vi "SELECT SALES TRACKING COLUMNS.vi"(8 "Search Database Results":refnum<vi>, 9 "DATA IN":string[][](array[string]), 11 "Sales Tracking Column Selector":T1={"SALE ID #"=TRUE, "BYU ID CARD #"=TRUE, "Sale Description"=TRUE, "Grand Total"=TRUE, "SALE DATE"=TRUE, "ITEM DESCRIPTION"=TRUE, "ITEM QUANTITY"=TRUE, "ITEM UNIT PRICE"=TRUE, "ITEM TOTAL PRICE"=TRUE, "SALE SEMESTER"=TRUE}) -> (1 "HEADERS OUT":string[](array[string]), 3 "DATA OUT":string[][](array[string]))   [LabVIEW 2019]
uses:
  Controls/Column Names/Sales Tracking Column Names.ctl
  <vilib>/Utility/miscctls.llb/LVRowAndColumnTypeDef.ctl
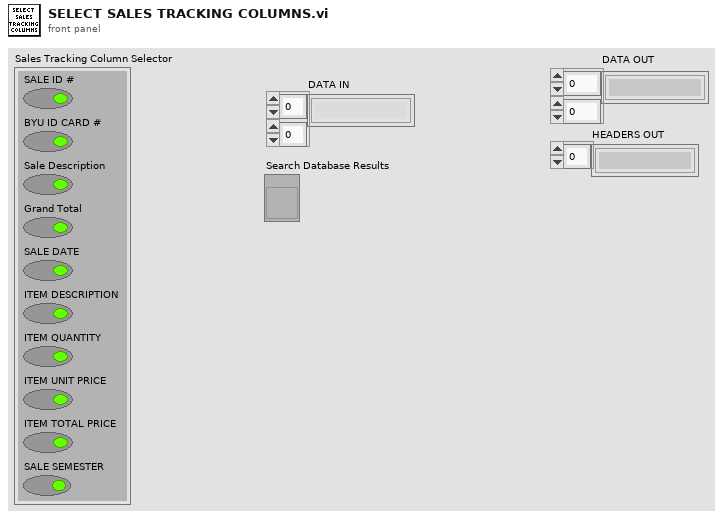
[diagram p1: front panel]
types:
  T1 = cluster{"SALE ID #":bool, "BYU ID CARD #":bool, "Sale Description":bool, "Grand Total":bool, "SALE DATE":bool, "ITEM DESCRIPTION":bool, "ITEM QUANTITY":bool, "ITEM UNIT PRICE":bool, "ITEM TOTAL PRICE":bool, "SALE SEMESTER":bool}
  T2 = typedef "Sales Tracking Column Names.ctl" = string[]
  T3 = typedef "LVRowAndColumnTypeDef.ctl" = cluster{"Row":i32, "Column":i32}
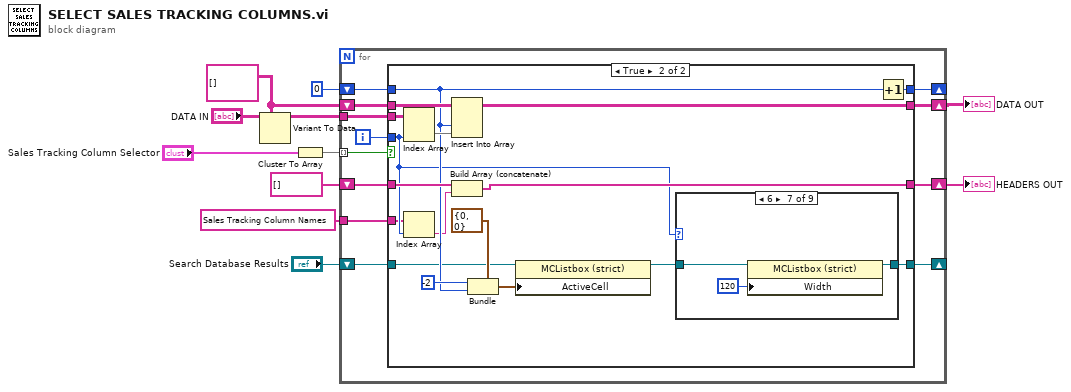
[diagram p0: block diagram]
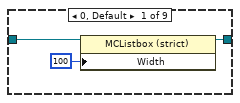
[diagram p3: hidden frame]
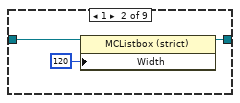
[diagram p4: hidden frame]
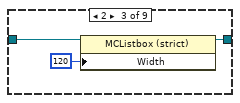
[diagram p5: hidden frame]
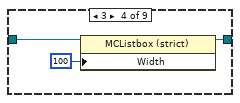
[diagram p6: hidden frame]
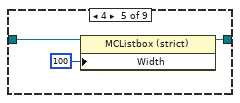
[diagram p7: hidden frame]
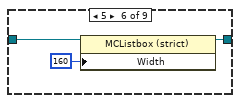
[diagram p8: hidden frame]
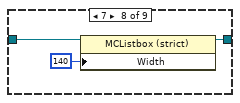
[diagram p9: hidden frame]
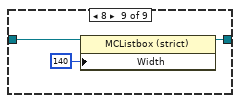
[diagram p10: hidden frame]
diagram:
  w7 = string[][] [] ("DATA OUT")
  n1 = Variant To Data(type=w7, Variant="DATA IN") -> (data=w8:string[][])  [unwired: 1 in, 1 out]
  n2 = Cluster To Array(cluster="Sales Tracking Column Selector") -> (array=w4:bool[])
  n3 = for {
    tunnel: w4 -> [w21] mode=indexing
    tunnel: w8 -> [w23]
    shift-right: [w17] -> w10
    shift-left: w7 -> [w20]
    shift-right: [w18] -> _
    shift-left: 0 -> [w19]
    shift-right: [w15] -> w9
    shift-left: string[] [] ("DATA OUT") -> [w16]
    shift-right: [w13] -> _
    shift-left: "Search Database Results" -> [w14]
    tunnel: T2 ["\"SALE ID #\"", "\"BYU ID CARD #\"", "\"Sale Description\"", "\"Grand Total\"", "\"Sale Date\"", "\"Item Description\"", "\"Item Quantity\"", "\"Item Unit Price\"", "\"Item Total Price\"", "\"Sale Semester\""] ("Sales Tracking Column Names") -> [w12]
    i -> [w22]
    n4 = case shown="True" w21 {
      tunnel: w23 -> [_ w44]
      tunnel: w22 -> [_ w31]
      tunnel: w20 -> [w26 w43]
      tunnel: w19 -> [w27 w34]
      tunnel: [w27 w41] -> w18
      tunnel: [w26 w40] -> w17
      tunnel: w16 -> [w25 w39]
      tunnel: [w25 w38] -> w15
      tunnel: w14 -> [w24 w33]
      tunnel: [w24 w30] -> w13
      tunnel: w12 -> [_ w29]
      frame False {
      }
      frame True {
        n5 = Index Array(array=w44, index (col)=w31) -> (element=w42:string[])  [unwired: 1 in]
        n6 = Index Array(array=w29, index=w31) -> (element=w28:string)
        n7 = Insert Into Array(array=w43, index (col)=w34, new element=w42) -> (w40:string[][])  [unwired: 1 in]
        n8 = Build Array (concatenate)(w39, w28) -> (w38:string[])
        n9 = Bundle(cluster=T3 {"Row"=0, "Column"=0} ("Active Cell:Active Cell"), "Row"=-2, "Column"=w34) -> (w37:T3)
        n10 = property class="MCListbox (strict)"(reference=w33, "ActiveCell"=w37) -> (reference out=w32:refnum<vi>)  [unwired: 1 in, 1 out]
        n11 = case shown="6" w31 {
          tunnel: w32 -> [w47 w50 w53 w56 w59 w62 w65 w68 w71]
          tunnel: [w46 w49 w52 w55 w58 w61 w64 w67 w70] -> w30
          frame 0, Default {
            n12 = property class="MCListbox (strict)"(reference=w47, "Width"=u32 100 ("Active Cell:Cell Size:Width")) -> (reference out=w46:refnum<vi>)  [unwired: 1 in, 1 out]
          }
          frame 1 {
            n13 = property class="MCListbox (strict)"(reference=w50, "Width"=u32 120 ("Active Cell:Cell Size:Width")) -> (reference out=w49:refnum<vi>)  [unwired: 1 in, 1 out]
          }
          frame 2 {
            n14 = property class="MCListbox (strict)"(reference=w53, "Width"=u32 120 ("Active Cell:Cell Size:Width")) -> (reference out=w52:refnum<vi>)  [unwired: 1 in, 1 out]
          }
          frame 3 {
            n15 = property class="MCListbox (strict)"(reference=w56, "Width"=u32 100 ("Active Cell:Cell Size:Width")) -> (reference out=w55:refnum<vi>)  [unwired: 1 in, 1 out]
          }
          frame 4 {
            n16 = property class="MCListbox (strict)"(reference=w59, "Width"=u32 100 ("Active Cell:Cell Size:Width")) -> (reference out=w58:refnum<vi>)  [unwired: 1 in, 1 out]
          }
          frame 5 {
            n17 = property class="MCListbox (strict)"(reference=w62, "Width"=u32 160 ("Active Cell:Cell Size:Width")) -> (reference out=w61:refnum<vi>)  [unwired: 1 in, 1 out]
          }
          frame 6 {
            n18 = property class="MCListbox (strict)"(reference=w65, "Width"=u32 120 ("Active Cell:Cell Size:Width")) -> (reference out=w64:refnum<vi>)  [unwired: 1 in, 1 out]
          }
          frame 7 {
            n19 = property class="MCListbox (strict)"(reference=w68, "Width"=u32 140 ("Active Cell:Cell Size:Width")) -> (reference out=w67:refnum<vi>)  [unwired: 1 in, 1 out]
          }
          frame 8 {
            n20 = property class="MCListbox (strict)"(reference=w71, "Width"=u32 140 ("Active Cell:Cell Size:Width")) -> (reference out=w70:refnum<vi>)  [unwired: 1 in, 1 out]
          }
        }
        n21 = Increment(x=w34) -> (x+1=w41:i32)
      }
    }
  }
  "DATA OUT" <- w10
  "HEADERS OUT" <- w9
